vi "Process State(Read Queue).vi"(0 "Process In":refnum<class "Process.lvclass">, 1 "Timeout in ms (-1)":i32, 11 "Error In":errorcluster) -> (4 "Process Out":refnum<class "Process.lvclass">, 8 "Message":T1, 10 "Timed Out?":bool, 15 "Error Out":errorcluster)   [LabVIEW 2023, in "Process.lvclass"]
doc: "Method encapsulating Read Queue state of process."
uses:
  Process.lvclass
  Interfaces/ICanCommunicate/Message.ctl
  Process.lvclass/Process.ctl
  Interfaces/ICanCommunicate/ICanCommunicate.lvclass
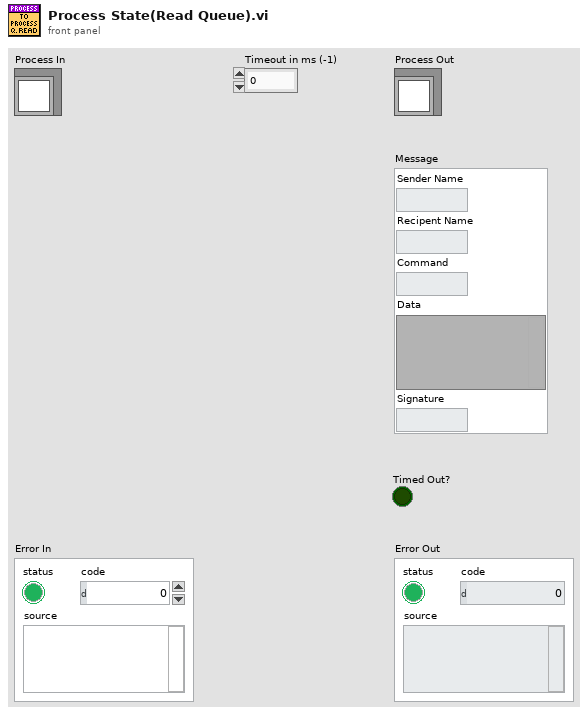
[diagram p1: front panel]
types:
  T1 = typedef "ICanCommunicate.lvclass/Message.ctl" = cluster{"Sender Name":string, "Recipent Name":string, "Command":string, "Data":variant, "Signature":string}
  T2 = typedef "ICanCommunicate.lvclass/ToProcessQueue.ctl" = refnum<queue>
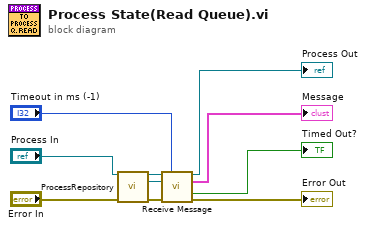
[diagram p0: block diagram]
diagram:
  n1 = call-dynamic "ProcessRepository.vi"("Process In"="Process In", "Error In"="Error In") -> ("Process Out"=w9:refnum<class "Process.lvclass">, "ToProcessQueue"=w8:T2, "Error Out"=w7:errorcluster)  [unwired: 7 in, 4 out]
  n2 = call-dynamic "Receive Message.vi"("ICanCommunicate In"=w9, "Timeout in ms (-1)"="Timeout in ms (-1)", "ToProcessQueue"=w8, "Error In"=w7) -> ("ICanCommunicate Out"=→"Process Out":refnum<class "Process.lvclass">, "Message"=→"Message":T1, "Timed Out?"=→"Timed Out?":bool, "Error Out"=→"Error Out":errorcluster)  [unwired: 8 in]
